vi "Selector.vi"(7 "Name":string="Selector", 11 "Nodes":refnum<class "abs_Node.lvclass">[](array[class])) -> (3 "Node":refnum<class "abs_Node.lvclass">)   [LabVIEW 2021, in "BT.lvlib"]
uses:
  BT.lvlib
  Support/Selector/Selector.lvclass
  C:/Users/Tim/Documents/GitHub/LV_Behaviour_Tree/Source/Support/abs_Composite/abs_Composite.lvclass
  C:/Users/Tim/Documents/GitHub/LV_Behaviour_Tree/Source/Support/abs_Node/abs_Node.lvclass
  C:/Program Files (x86)/National Instruments/LabVIEW 2021/vi.lib/TSA/Abstract Data Classes/Abs_Types/Type/Abs_Type.lvclass
  C:/Users/Tim/Documents/GitHub/LV_Behaviour_Tree/Source/Support/Selector/Selector.lvclass
  Support/abs_Node/abs_Node.lvclass
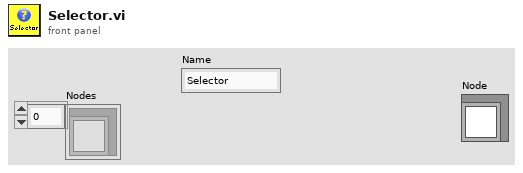
[diagram p1: front panel]
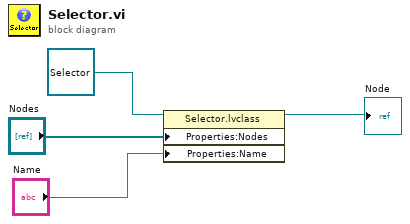
[diagram p0: block diagram]
diagram:
  n1 = property class="Selector.lvclass"(reference=refnum<class "Selector.lvclass"> refnum ("BT.lvlib:Selector.lvclass"), "Properties:Nodes"="Nodes", "Properties:Name"="Name") -> (reference out=→"Node":refnum<class "Selector.lvclass">)  [unwired: 1 in, 1 out]
